vi "Create File with Incrementing Suffix Fast.vi"(6 "disable buffering (F)":bool, 7 "format string (\" (%d)\")":string=" (%d)", 8 "error in (no error)":errorcluster, 11 "file path":path) -> (0 "error out":errorcluster, 2 "actual path":path, 3 "refnum out":refnum<file>)   [LabVIEW 2016]
doc: "Creates a file and appends an incrementing number suffix to the filename if the file already exists at a specified path. If the file does not exist, this VI creates the file without appending an incrementing number suffix to the filename."
panel:
  out "x-y":dbl
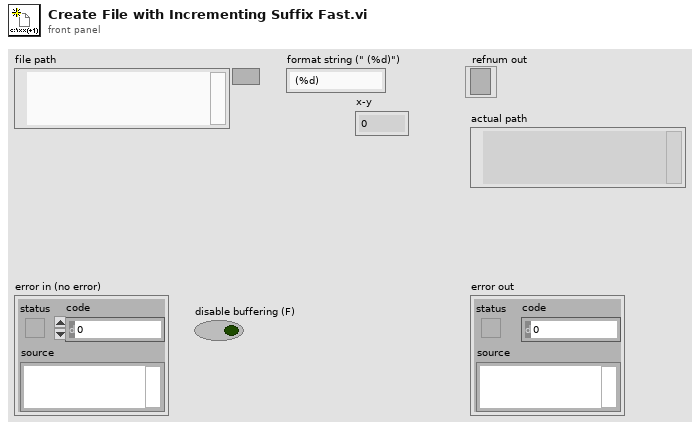
[diagram p1: front panel]
types:
  T1 = enum16{"open", "replace", "create", "open or create", "replace or create", "replace or create with confirmation"}
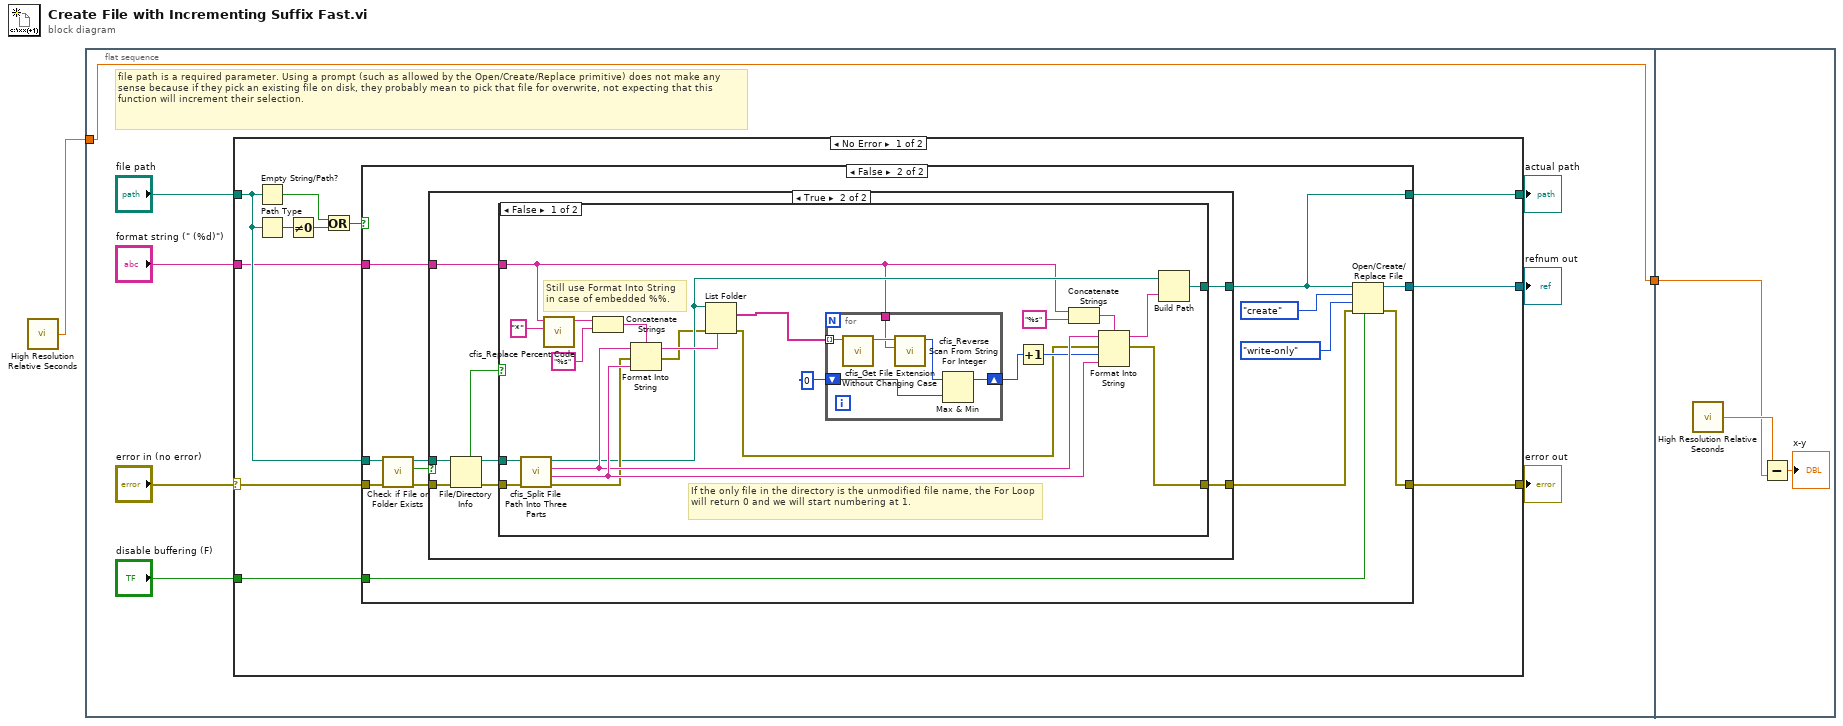
[diagram p0: block diagram]
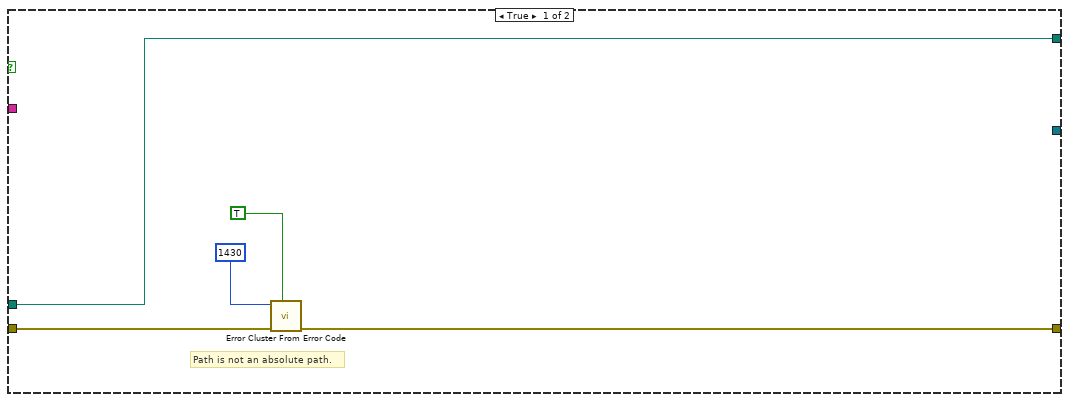
[diagram p2: hidden frame]
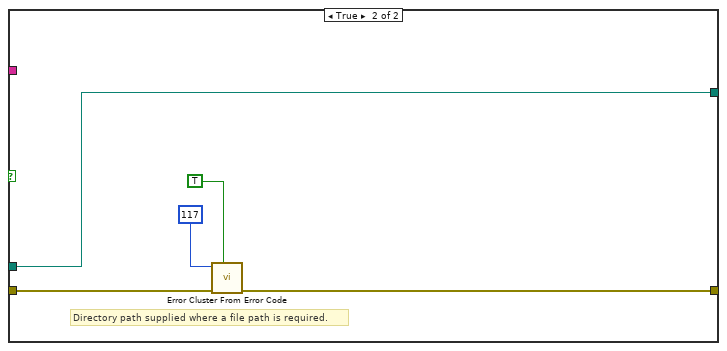
[diagram p4: hidden frame]
diagram:
  n1 = call <vilib>:"High Resolution Relative Seconds.vi"() -> ("relative seconds"=w1:dbl)
  n2 = flat-sequence {
    tunnel: [w3] -> w2
    tunnel: w1 -> [w3]
    tunnel: w2 -> [w86]
    frame #0 {
      # "file path is a required parameter. Using a prompt (such as allowed by the Open/Create/Replace primitive) does not make any sense because if they pick an existing file on disk, they probably mean to pick that file for overwrite, not expecting that this function will increment their selection."
      n3 = case shown="No Error" "error in (no error)" {
        selector: "error in (no error)" -> [w18 w84]
        tunnel: "file path" -> [w13 w83]
        tunnel: "disable buffering (F)" -> [w21 _]
        tunnel: [w20 w84] -> w8
        tunnel: [w19 _] -> w7
        tunnel: [w12 w83] -> w5
        tunnel: "format string (\" (%d)\")" -> [w11 _]
        frame No Error {
          n4 = Empty String/Path?(string/path=w13) -> (empty?=w15:bool)
          n5 = Path Type(1:w13) -> (0:w17:i16)
          n6 = Not Equal To 0?(x=w17) -> (x != 0?=w16:bool)
          n7 = Or(x=w15, y=w16) -> (x .or. y?=w14:bool)
          n8 = case shown="False" w14 {
            tunnel: w21 -> [_ w39]
            tunnel: [w26 w38] -> w20
            tunnel: [_ w37] -> w19
            tunnel: w18 -> [w24 w36]
            tunnel: w13 -> [w22 w35]
            tunnel: [w22 w28] -> w12
            tunnel: w11 -> [_ w27]
            frame True {
              # "Path is not an absolute path."
              n9 = call <vilib>:"Error Cluster From Error Code.vi"("show call chain? (False)"=TRUE, "error in (no error)"=w24, "error code (0)"=1430) -> ("error out"=w26:errorcluster)  [unwired: 6 in]
            }
            frame False {
              n10 = call <vilib>:"Check if File or Folder Exists.vi"("error in (no error)"=w36, "path"=w35) -> ("error out"=w30:errorcluster, "file or folder exists?"=w32:bool, "dup path"=w31:path)  [unwired: 7 in]
              n11 = case shown="True" w32 {
                tunnel: w31 -> [w41 w49]
                tunnel: [w41 w43] -> w28
                tunnel: w30 -> [w40 w48]
                tunnel: [w40 w45] -> w29
                tunnel: w27 -> [_ w42]
                frame False {
                }
                frame True {
                  n12 = File/Directory Info(path=w49, error in=w48) -> (path out=w44:path, directory=w47:bool, error out=w46:errorcluster)  [unwired: 4 out]
                  n13 = case shown="False" w47 {
                    tunnel: w46 -> [w62 w82]
                    tunnel: [w55 w79] -> w45
                    tunnel: w44 -> [w71 w78]
                    tunnel: [w56 w78] -> w43
                    tunnel: w42 -> [w53 _]
                    frame False {
                      # "If the only file in the directory is the unmodified file name, the For Loop will return 0 and we will start numbering at 1."
                      # "Still use Format Into String\nin case of embedded %%."
                      n14 = call <vilib>:"cfis_Split File Path Into Three Parts.vi"("file path"=w71) -> ("File extension"=w64:string, "File name without extension"=w63:string, "Directory"=w60:path)  [unwired: 8 in]
                      n15 = call <vilib>:"cfis_Replace Percent Code.vi"("replace text"="*", "format string in"=w53) -> ("format string out"=w67:string)  [unwired: 9 in]
                      n16 = Concatenate Strings(w67, "%s" ("format string")) -> (w66:string)
                      n17 = Format Into String(format string=w66, initial string=w63, error in=w62, w64) -> (resulting string=w61:string, error out=w59:errorcluster)
                      n18 = List Folder(path=w60, pattern=w61, error in=w59) -> (filenames=w51:string[], error out=w54:errorcluster)  [unwired: 1 in, 2 out]
                      n19 = for {
                        tunnel: w51 -> [w77] mode=indexing
                        shift-right: [w73] -> w50
                        shift-left: 0 -> [w74]
                        tunnel: w53 -> [w72]
                        n20 = call <vilib>:"cfis_Get File Extension Without Changing Case.vi"("file name"=w77) -> ("file name without extension"=w76:string)  [unwired: 9 in, 1 out]
                        n21 = call <vilib>:"cfis_Reverse Scan From String For Integer.vi"("format string"=w72, "input string"=w76) -> ("Extracted integer"=w75:i32)  [unwired: 9 in]
                        n22 = Max & Min(x=w75, y=w74) -> (max(x,y)=w73:i32)  [unwired: 1 out]
                      }
                      n23 = Increment(x=w50) -> (x+1=w57:i32)
                      n24 = Concatenate Strings(w53, "%s" ("format string")) -> (w69:string)
                      n25 = Format Into String(format string=w69, initial string=w63, error in=w54, w57, w64) -> (resulting string=w58:string, error out=w55:errorcluster)
                      n26 = Build Path(base path=w60, name or relative path=w58) -> (appended path=w56:path)
                    }
                    frame True {
                      # "Directory path supplied where a file path is required."
                      n27 = call <vilib>:"Error Cluster From Error Code.vi"("show call chain? (False)"=TRUE, "error in (no error)"=w82, "error code (0)"=117) -> ("error out"=w79:errorcluster)  [unwired: 6 in]
                    }
                  }
                }
              }
              n28 = Open/Create/Replace File(file path (use dialog)=w28, error in=w29, operation (0:open)=T1."create", access (0:read/write)=enum16{"read/write", "read-only", "write-only"}."write-only", disable buffering (F)=w39) -> (refnum out=w37:refnum<file>, error out=w38:errorcluster)  [unwired: 1 in, 1 out]
            }
          }
        }
        frame Error {
        }
      }
      "error out" <- w8
      "refnum out" <- w7
      "actual path" <- w5
    }
    frame #1 {
      n29 = call <vilib>:"High Resolution Relative Seconds.vi"() -> ("relative seconds"=w87:dbl)
      n30 = Subtract(x=w87, y=w86) -> (x-y=→"x-y":dbl)
    }
  }
